vi "calcolo compensazione C.vi"(0 "P imp":dbl, 1 "C max freno [n/m]":dbl=2120.0, 5 "P resa letta":dbl, 7 "RPM nom":dbl, 9 "RPM":dbl, 11 "precisione kw":dbl) -> (6 "C [Nm]":dbl, 10 "Precisione C[Nm]":dbl)   [LabVIEW 2019]
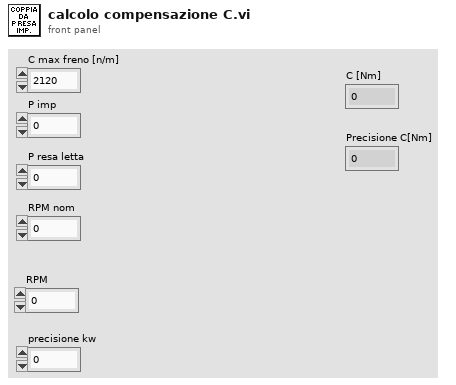
[diagram p1: front panel]
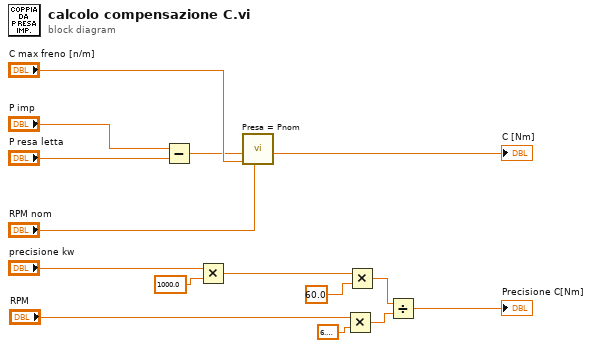
[diagram p0: block diagram]
diagram:
  n1 = Subtract(x="P imp", y="P resa letta") -> (x-y=w4:dbl)
  n2 = Multiply(x="precisione kw", y=1000.0) -> (x*y=w1:dbl)
  n3 = call "Presa = Pnom.vi"("RPM nom"="RPM nom", "C max freno [n/m]"="C max freno [n/m]", "P imp (kw)"=w4) -> ("C [Nm]"=→"C [Nm]":dbl)  [unwired: 7 in, 1 out]
  n4 = Multiply(x="RPM", y=6.283185307179586) -> (x*y=w6:dbl)
  n5 = Multiply(x=w1, y=60.0) -> (x*y=w9:dbl)
  n6 = Divide(x=w9, y=w6) -> (x/y=→"Precisione C[Nm]":dbl)
